vi "Close Download Task.vi"(8 "error in (no error)":errorcluster, 11 "HttpDownloadTask in":T1) -> (0 "error out":errorcluster)   [LabVIEW 2018, in "LabVIEWHTTPClient_NET.lvlib" / "HttpDownloadTask.lvclass"]
uses:
  HttpDownloadTask.lvclass
  Types/DownloadTask_ref.ctl
  HttpDownloadTask.lvclass/HttpDownloadTask.ctl
  HttpContent/HttpContent.lvclass
  HttpResponseMessage/HttpResponseMessage.lvclass
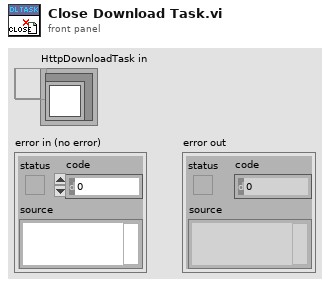
[diagram p1: front panel]
types:
  T1 = typedef "LabVIEWHTTPClient_NET.lvlib/HttpDownloadTask.lvclass/DownloadTask_ref.ctl" = refnum<data-value>
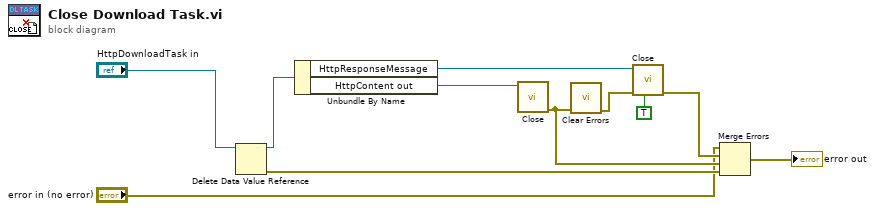
[diagram p0: block diagram]
diagram:
  n1 = Delete Data Value Reference(data value reference="HttpDownloadTask in") -> (data value=w10:refnum<class "HttpDownloadTask.lvclass">, error out=w3:errorcluster)  [unwired: 1 in]
  n2 = Unbundle By Name(w10) -> ("HttpResponseMessage"=w7:refnum<class "HttpResponseMessage.lvclass">, "HttpContent out"=w8:refnum<class "HttpContent.lvclass">)
  n3 = call "Close.vi"("HttpContent in"=w8) -> ("error out"=w5:errorcluster)  [unwired: 10 in]
  n4 = call <vilib>:"Clear Errors.vi"("error in (no error)"=w5) -> ("error out"=w4:errorcluster)  [unwired: 5 in, 1 out]
  n5 = call "Close.vi"("CloseHeaders"=TRUE, "error in (no error)"=w4, "HttpResponseMessage in"=w7) -> ("error out"=w6:errorcluster)  [unwired: 8 in]
  n6 = Merge Errors("error in (no error)", w6, w5, w3) -> (→"error out":errorcluster)
